vi "Freemailemailkliens .vi"() -> ()   [LabVIEW 2020]
uses:
  <vilib>/smtpClient/Set Message Text.vi
  <vilib>/smtpClient/LabVIEWSMTPClient.lvlib
panel:
  in  "attachments":path[](array[path])
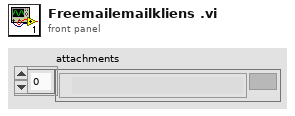
[diagram p1: front panel]
types:
  T1 = typedef "LabVIEWSMTPClient.lvlib/SmtpClientHandle.ctl" = refnum<k1>
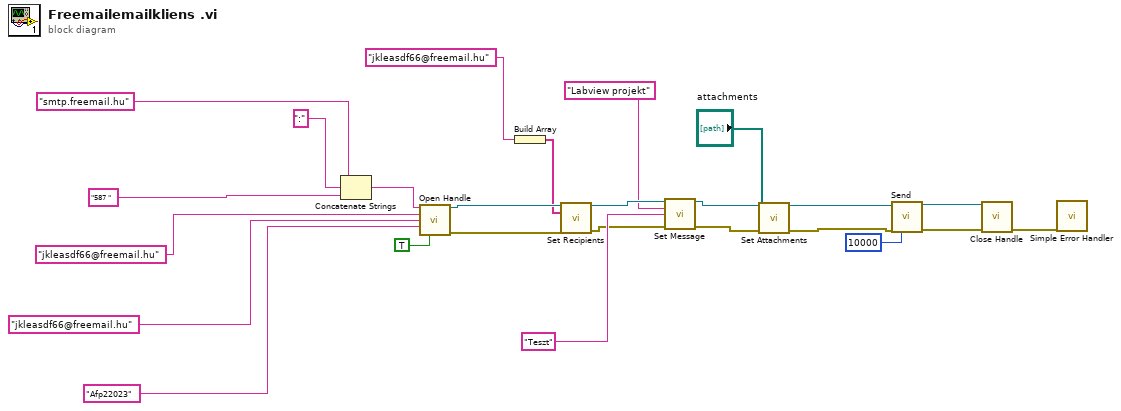
[diagram p0: block diagram]
diagram:
  n1 = Concatenate Strings("smtp.freemail.hu" ("string"), ":" ("string"), "587 " ("string")) -> (w22:string)
  n2 = call <vilib>:"Open Handle.vi"("server address"=w22, "from"="jkleasdf66@freemail.hu" ("username"), "username"="jkleasdf66@freemail.hu", "password"="Afp22023", "use TLS (false)"=TRUE) -> ("handle out"=w25:T1, "error out"=w8:errorcluster)  [unwired: 9 in]
  n3 = Build Array("jkleasdf66@freemail.hu" ("username")) -> (w20:string[])
  n4 = call <vilib>:"Set Recipients.vi"("handle in"=w25, "to"=w20, "error in (no error)"=w8) -> ("handle out"=w24:T1, "error out"=w7:errorcluster)  [unwired: 11 in]
  n5 = call-poly <vilib>:"Set Message.vi"("handle in"=w24, "subject"="Labview projekt", "plain text message"="Teszt", "error in (no error)"=w7) -> ("handle out"=w10:T1, "error out"=w6:errorcluster)  [unwired: 10 in]
  n6 = call <vilib>:"Set Attachments.vi"("handle in"=w10, "attachments"="attachments", "error in (no error)"=w6) -> ("handle out"=w9:T1, "error out"=w5:errorcluster)  [unwired: 11 in]
  n7 = call <vilib>:"Send.vi"("handle in"=w9, "error in (no error)"=w5, "timeout in ms (10000)"=10000) -> ("handle out"=w23:T1, "error out"=w4:errorcluster)  [unwired: 10 in, 1 out]
  n8 = call <vilib>:"Close Handle.vi"("handle in"=w23, "error in (no error)"=w4) -> ("error out"=w2:errorcluster)  [unwired: 12 in, 1 out]
  n9 = call <vilib>:"Simple Error Handler.vi"("error in (no error)"=w2) -> ()  [unwired: 4 in, 5 out]
